vi "Index By Pressure.vi"(1 "Air Pressure [psia]":dbl) -> (0 "Pressure Index":dbl)   [LabVIEW 2020]
uses:
  <vilib>/gmath/NI_Gmath.lvlib
panel:
  out "Pressure Used":dbl[](array[numeric]) format="%_6g"
  in  "Pressure Array":dbl[](array[numeric])=[15.51026974, 15.23488864, 14.96348006, 14.696, 14.43240481, 14.17265118, 13.91669613, 13.66449702, 13.41601153, 13.17119769, 12.93001384, 12.69241866, 12.45837117, 12.22783068, 12.00075687, 11.77710969, 11.55684946, 11.3399368]
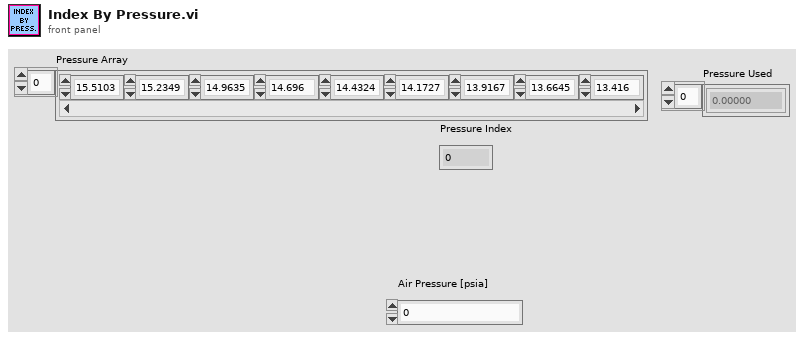
[diagram p1: front panel]
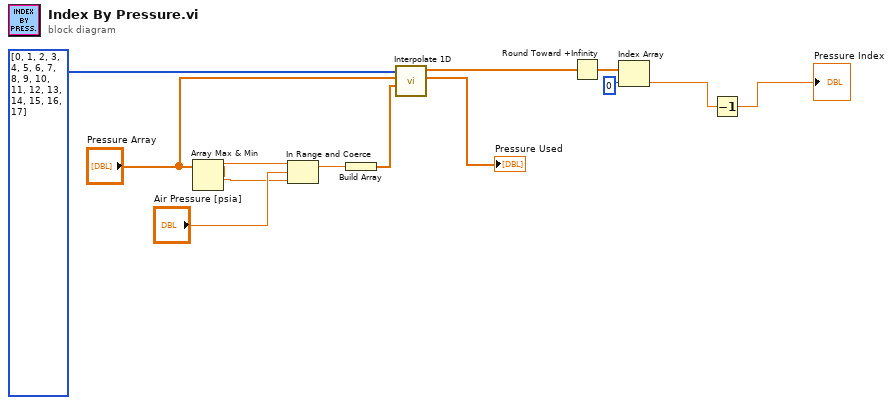
[diagram p0: block diagram]
diagram:
  n1 = Array Max & Min(array="Pressure Array") -> (max value=w8:dbl, min value=w7:dbl)  [unwired: 2 out]
  n2 = In Range and Coerce(upper limit=w8, x="Air Pressure [psia]", lower limit=w7) -> (coerced(x)=w6:dbl)  [unwired: 1 out]
  n3 = Build Array(w6) -> (w12:dbl[])
  n4 = call <vilib>:"Interpolate 1D.vi"("xi"=w12, "X"="Pressure Array", "Y"=i32[] [0, 1, 2, 3, 4, 5, 6, 7, 8, 9, 10, 11, 12, 13, 14, 15, 16, 17]) -> ("xi used"=→"Pressure Used":dbl[], "yi"=w11:dbl[])  [unwired: 6 in, 1 out]
  n5 = Round Toward +Infinity(x=w11) -> (ceil(x): smallest int >= x=w3:dbl[])
  n6 = Index Array(array=w3, index=0) -> (element=w2:dbl)
  n7 = Decrement(x=w2) -> (x-1=→"Pressure Index":dbl)
